vi "build_color-markers.vi"(11 "images":dbl[][][](array[numeric])) -> (3 "color_markers":cluster{dbl, u32}[](array[cluster]))   [LabVIEW 2018]
panel:
  out "image":dbl[][](graph)
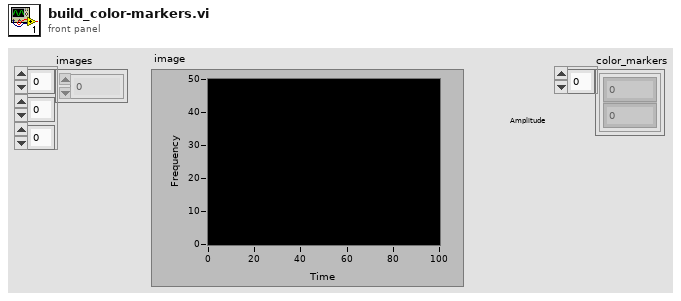
[diagram p1: front panel]
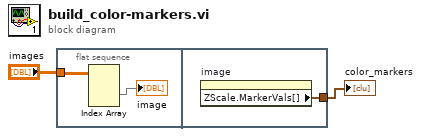
[diagram p0: block diagram]
diagram:
  n1 = flat-sequence {
    tunnel: "images" -> [w3]
    tunnel: [w5] -> w1
    frame #0 {
      n2 = Index Array(array=w3) -> (element=→"image":dbl[][])  [unwired: 3 in]
    }
    frame #1 {
      n3 = property on="image" class="IntGraph (strict)"() -> ("ZScale.MarkerVals[]"=w5:cluster{dbl, u32}[])  [unwired: 2 in, 2 out]
    }
  }
  "color_markers" <- w1
